vi "Capability Query.vi"(8 "error in (no error)":errorcluster) -> (0 "error out":errorcluster)   [LabVIEW 2020, in "FirmataClient.lvlib"]
doc: "Retrieve the capability of all the pins of the currently connected board. This mainly includes the list of modes supported by each pin along with the resolution for the mode (i.e. a Pin supporting Analog Mode might have a resolution of 14bits)"
uses:
  FirmataClient.lvlib
panel:
  in  "Queue Name":string="firmata-serial-communication"
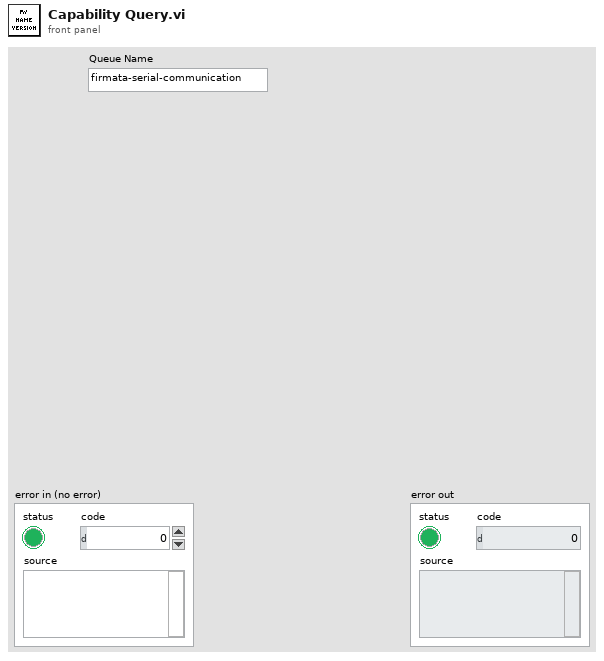
[diagram p1: front panel]
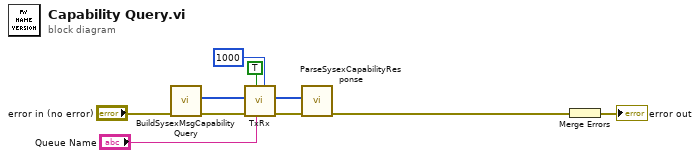
[diagram p0: block diagram]
diagram:
  n1 = call "BuildSysexMsgCapabilityQuery.vi"("error in"="error in (no error)") -> ("error out"=w2:errorcluster, "GetCapabilitiesMessage"=w3:u8[])  [unwired: 7 in, 2 out]
  n2 = call "TxRx.vi"("Reply Timeout Ms"=1000, "Queue Name"="Queue Name", "Wait For Reply?"=TRUE, "error in"=w2, "Message"=w3) -> ("error out"=w1:errorcluster, "Reply"=w4:u8[])  [unwired: 5 in]
  n3 = call "ParseSysexCapabilityResponse.vi"("error in"=w1, "Sysex Message"=w4) -> ("error out"=w9:errorcluster)  [unwired: 8 in, 1 out]
  n4 = Merge Errors(w9) -> (→"error out":errorcluster)
